vi "游标移动显示.vi"(4 "偏移值":i32, 6 "游标位置":cluster{"X":dbl, "Y":dbl}, 7 "CursIdx":i32, 9 "游标文本":refnum<vi>, 10 "XYGraph":refnum<vi>, 11 "YBNum":refnum<vi>) -> ()   [LabVIEW 2015]
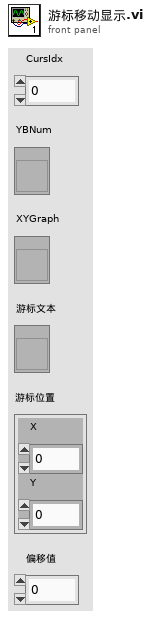
[diagram p1: front panel]
types:
  T1 = typedef "LVRectTypeDef.ctl" = cluster{"Left":i16, "Top":i16, "Right":i16, "Bottom":i16}
  T2 = typedef "LVPoint32TypeDef.ctl" = cluster{"Horizontal":i32, "Vertical":i32}
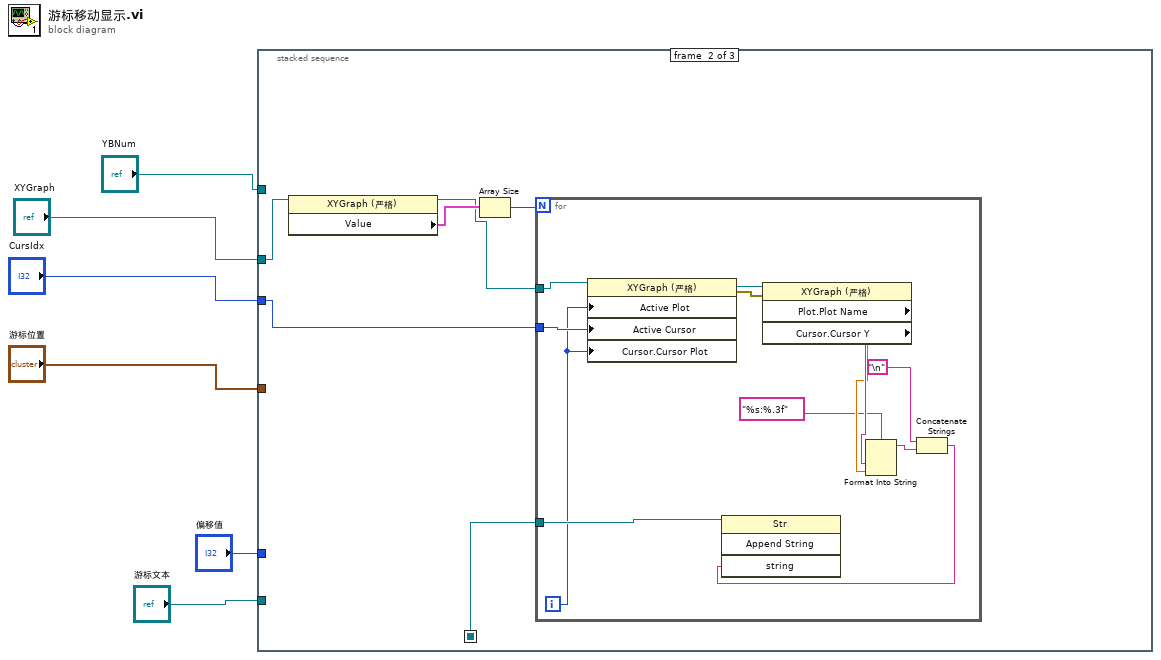
[diagram p0: block diagram]
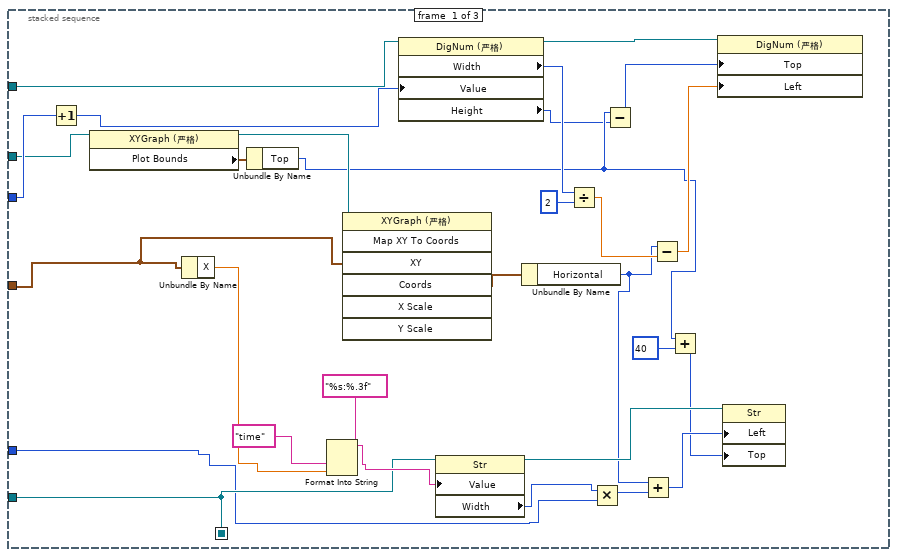
[diagram p2: hidden frame]
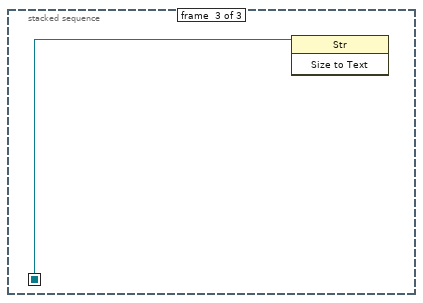
[diagram p3: hidden frame]
diagram:
  n1 = stacked-sequence {
    seq-local: [w14 _ _] -> [_ w36 w54]
    tunnel: "CursIdx" -> [w34 w37 _]
    tunnel: "游标位置" -> [w30 _ _]
    tunnel: "XYGraph" -> [w33 w41 _]
    tunnel: "YBNum" -> [w23 _ _]
    tunnel: "游标文本" -> [w14 _ _]
    tunnel: "偏移值" -> [w13 _ _]
    frame #0 {
      n2 = Increment(x=w34) -> (x+1=w12:i32)
      n3 = property class="XYGraph (严格)"(reference=w33) -> (reference out=w31:refnum<vi>, "Plot Bounds"=w32:T1)  [unwired: 1 in, 1 out]
      n4 = Unbundle By Name(w30) -> ("X"=w8:dbl)
      n5 = Unbundle By Name(w32) -> ("Top"=w10:i16)
      n6 = Format Into String(format string="%s:%.3f" ("格式字符串"), "time" ("格式字符串"), w8) -> (resulting string=w21:string)  [unwired: 2 in, 1 out]
      n7 = invoke class="XYGraph (严格)" method="Map XY To Coords"(reference=w31, "XY"=w30) -> ("Coords"=w28:T2)  [unwired: 5 in, 6 out]
      n8 = property class="DigNum (严格)"(reference=w23, "Value"=w12) -> (reference out=w29:refnum<vi>, "Width"=w24:u32, "Height"=w9:u32)  [unwired: 1 in, 1 out]
      n9 = property class="Str"(reference=w14, "Value"=w21) -> (reference out=w22:refnum<vi>, "Width"=w18:u32)  [unwired: 1 in, 1 out]
      n10 = Unbundle By Name(w28) -> ("Horizontal"=w19:i32)
      n11 = Divide(x=w24, y=u32 2) -> (x/y=w25:dbl)
      n12 = Multiply(x=w18, y=w13) -> (x*y=w20:u32)
      n13 = Subtract(x=w10, y=w9) -> (x-y=w11:u32)
      n14 = Add(x=w19, y=w20) -> (x+y=w17:u32)
      n15 = Subtract(x=w19, y=w25) -> (x-y=w27:dbl)
      n16 = Add(x=w10, y=i16 40) -> (x+y=w15:i16)
      n17 = property class="DigNum (严格)"(reference=w29, "Top"=w11, "Left"=w27) -> ()  [unwired: 1 in, 2 out]
      n18 = property class="Str"(reference=w22, "Left"=w17, "Top"=w15) -> ()  [unwired: 1 in, 2 out]
    }
    frame #1 {
      n19 = property class="XYGraph (严格)"(reference=w41) -> (reference out=w38:refnum<vi>, "Value"=w39:cluster{dbl[], dbl[]}[])  [unwired: 1 in, 1 out]
      n20 = Array Size(array=w39) -> (size(s)=w40:i32)
      n21 = for {
        N: w40 -> [_]
        tunnel: w36 -> [w51]
        tunnel: w37 -> [w49]
        tunnel: w38 -> [w43]
        i -> [w44]
        n22 = property class="XYGraph (严格)"(reference=w43, "Active Plot"=w44, "Active Cursor"=w49, "Cursor.Cursor Plot"=w44) -> (reference out=w48:refnum<vi>, error out=w47:errorcluster)  [unwired: 1 in]
        n23 = property class="XYGraph (严格)"(reference=w48, error in=w47) -> ("Plot.Plot Name"=w46:string, "Cursor.Cursor Y"=w45:dbl)  [unwired: 2 out]
        n24 = Format Into String(format string="%s:%.3f" ("格式字符串"), w46, w45) -> (resulting string=w53:string)  [unwired: 2 in, 1 out]
        n25 = Concatenate Strings("\n", w53) -> (w50:string)
        n26 = invoke class="Str" method="Append String"(reference=w51, "string"=w50) -> ()  [unwired: 2 in, 4 out]
      }
    }
    frame #2 {
      n27 = invoke class="Str" method="Size to Text"(reference=w54) -> ()  [unwired: 2 in, 3 out]
    }
  }
